vi "setOutputState.vi"(8 "error in (no error)":errorcluster, 10 "State":bool, 11 "VISA resource name":refnum<visa-resource-name>) -> (0 "error out":errorcluster, 3 "VISA resource name out":refnum<visa-resource-name>)   [LabVIEW 2023, in "Keysight-33500B.lvlib"]
doc: "<b>Author:</b> Wolfgang\n<b>Description:</b> >>>> Enable/Disable Output >>>"
uses:
  Keysight-33500B.lvlib
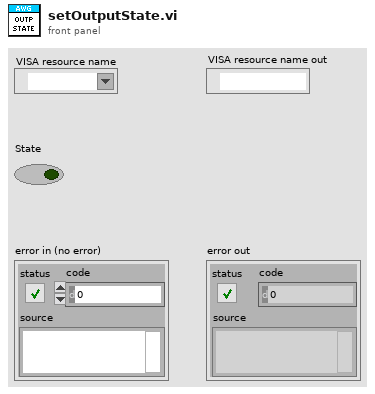
[diagram p1: front panel]
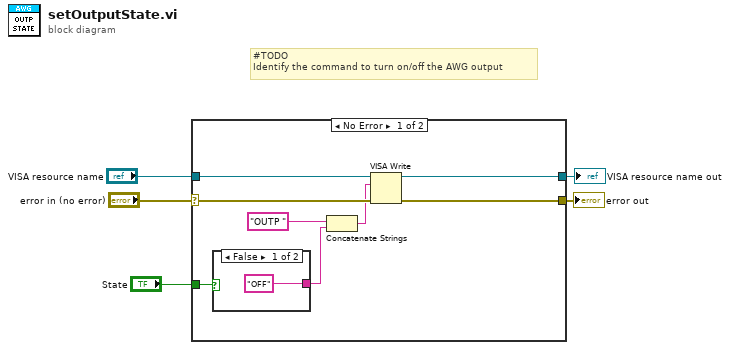
[diagram p0: block diagram]
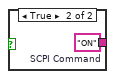
[diagram p2: hidden frame]
diagram:
  # "#TODO\nIdentify the command to turn on/off the AWG output"
  n1 = case shown="No Error" "error in (no error)" {
    selector: "error in (no error)" -> [w12 w17]
    tunnel: [w7 w16] -> w5
    tunnel: [w6 w17] -> w3
    tunnel: "VISA resource name" -> [w13 w16]
    tunnel: "State" -> [w8 _]
    frame No Error {
      n2 = case shown="False" w8 {
        tunnel: ["OFF" ("SCPI Command") w15] -> w9
        frame False {
        }
        frame True {
          w15 = "ON"  # SCPI Command
        }
      }
      n3 = Concatenate Strings("OUTP ", w9) -> (w10:string)
      n4 = VISA Write(VISA resource name=w13, write buffer=w10, error in (no error)=w12) -> (VISA resource name out=w7:refnum<visa-resource-name>, error out=w6:errorcluster)  [unwired: 1 out]
    }
    frame Error {
    }
  }
  "VISA resource name out" <- w5
  "error out" <- w3
